vi "test_write_SV.vi"() -> ()   [LabVIEW 2018]
panel:
  out "error out 2":errorcluster
  out "error out":errorcluster
  in  "stop":bool
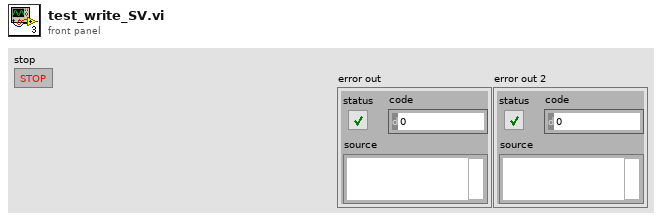
[diagram p1: front panel]
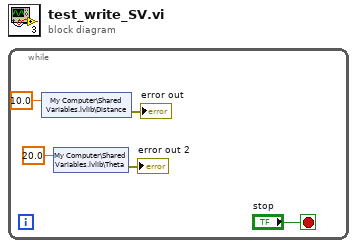
[diagram p0: block diagram]
diagram:
  n1 = while {
    stop <- "stop" stop-if-true
    n2 = shared-variable "My Computer\\Shared Variables.lvlib\\Distance"(10.0 ("Distance")) -> (error out=→"error out":errorcluster)  [unwired: 1 in]
    n3 = shared-variable "My Computer\\Shared Variables.lvlib\\Theta"(20.0 ("Theta")) -> (error out=→"error out 2":errorcluster)  [unwired: 1 in]
  }
